vi "Export_2DtoTxt.vi"(2 "Auto?":bool, 3 "Data (2D)":dbl[][](array[numeric]), 4 "Export Type":string, 5 "Filename":string) -> ()   [LabVIEW 2010]
uses:
  <vilib>/Utility/file.llb/Write To Spreadsheet File (DBL).vi
panel:
  out "File Path":path
  in  "Auto Folder":path caption="Ausgewählter Pfad"
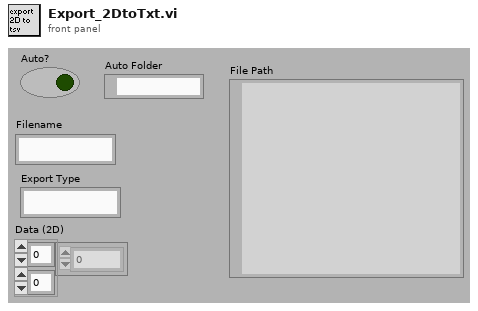
[diagram p1: front panel]
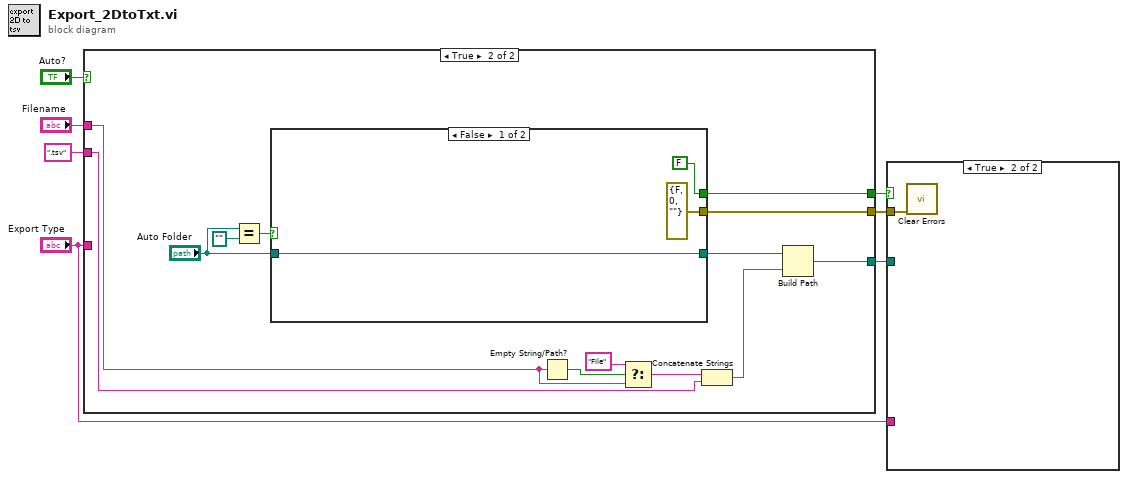
[diagram p0: block diagram]
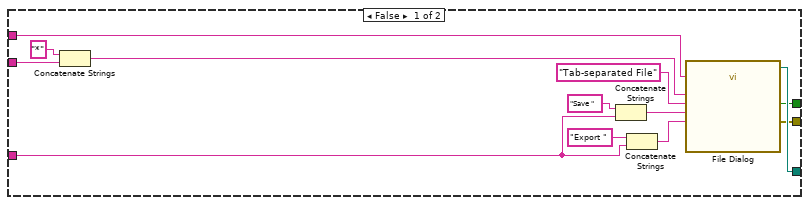
[diagram p2: hidden frame]
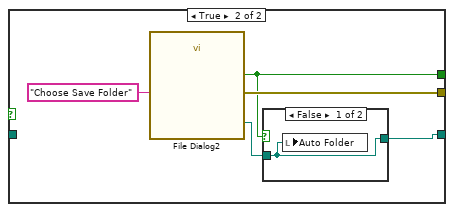
[diagram p3: hidden frame]
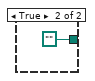
[diagram p4: hidden frame]
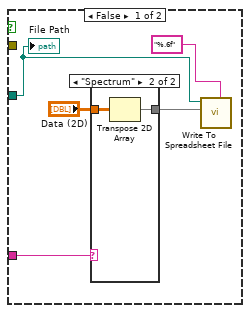
[diagram p5: hidden frame]
diagram:
  n1 = case shown="True" "Auto?" {
    tunnel: "Export Type" -> [w15 _]
    tunnel: [w14 w27] -> w5
    tunnel: [w13 w25] -> w4
    tunnel: [w12 w26] -> w3
    tunnel: ".tsv" ("pattern (all files)") -> [w10 w33]
    tunnel: "Filename" -> [w11 w23]
    frame False {
      n2 = Concatenate Strings("*" ("String"), w10) -> (w8:string)
      n3 = Concatenate Strings("Save " ("prompt"), w15) -> (w20:string)
      n4 = Concatenate Strings("Export " ("button label"), w15) -> (w19:string)
      n5 = call "File Dialog"("prompt"=w19, "button label"=w20, "default name"=w11, "pattern (all files)"=w8, "pattern label"="Tab-separated File") -> ("selected path"=w14:path, "cancelled"=w13:bool, "error out"=w12:errorcluster)  [unwired: 7 in, 1 out]
    }
    frame True {
      n6 = Equal?(x="Auto Folder", y=path "") -> (x = y?=w30:bool)
      n7 = case shown="False" w30 {
        tunnel: "Auto Folder" -> [w36 _]
        tunnel: [w36 w40] -> w32
        tunnel: [errorcluster {"status"=FALSE, "code"=0, "source"=""} ("error out") w39] -> w26
        tunnel: [FALSE ("cancelled") w38] -> w25
        frame False {
        }
        frame True {
          n8 = call "File Dialog2"("prompt"="Choose Save Folder") -> ("selected path"=w41:path, "cancelled"=w38:bool, "error out"=w39:errorcluster)  [unwired: 11 in, 1 out]
          n9 = case shown="False" w38 {
            tunnel: w41 -> [w42 _]
            tunnel: [w42 path ""] -> w40
            frame False {
              n10 = local write "Auto Folder"(w42) -> ()
            }
            frame True {
            }
          }
        }
      }
      n11 = Empty String/Path?(string/path=w23) -> (empty?=w24:bool)
      n12 = Select(t="File", s=w24, f=w23) -> (s? t:f=w21:string)
      n13 = Concatenate Strings(w21, w33) -> (w28:string)
      n14 = Build Path(base path=w32, name or relative path=w28) -> (appended path=w27:path)
    }
  }
  n15 = case shown="True" w4 {
    tunnel: w5 -> [w45 _]
    tunnel: w3 -> [_ w52]
    tunnel: "Export Type" -> [w46 _]
    frame False {
      n16 = case shown="\"Spectrum\"" w46 {
        tunnel: "Data (2D)" -> [w49 w51]
        tunnel: [w49 w50] -> w47
        frame "Map", Default {
        }
        frame "Spectrum" {
          n17 = Transpose 2D Array(2D array=w51) -> (transposed array=w50:dbl[][])
        }
      }
      n18 = call-poly <vilib>:"Write To Spreadsheet File.vi"("format (%.3f)"="%.6f", "2D data"=w47, "file path (dialog if empty)"=w45) -> ()  [unwired: 5 in, 1 out]
      "File Path" <- w45
    }
    frame True {
      n19 = call <vilib>:"Clear Errors.vi"("error in (no error)"=w52) -> ()  [unwired: 6 in, 1 out]
    }
  }
